vi "FCE_TS_Action_WriteChannelNames.vi"() -> ()   [LabVIEW 2017]
uses:
  FCE_TS_FGlob_V001.llb/FCE_TS_FGlob_TDefEnumcDAQDIItems.ctl
  FCE_TS_FGlob_V001.llb/FCE_TS_FGlob_TDefEnumcDAQDOItems.ctl
  FCE_TS_FGlob_V001.llb/FCE_TS_FGlob_TDefEnumcDAQAIItems.ctl
  FCE_TS_FGlob_V001.llb/FCE_TS_FGlob_TDefEnumcDAQAOItems.ctl
  FCE_TS_FGlob_V001.llb/FCE_TS_FGlob_TDefEnumCANReadItems.ctl
panel:
  in  "Tab Control":enum32{"DI", "DO", "AI", "AO", "CAN"}(tab)
  in  "PCI DI Item":T1
  out "Signal Name":string[](array[string])=["EK_TS", "EZ_Um1", "EZ_Um2", "EZ_Um3", "WZ_TS", "NP", "LP", "HP", "ROP", "CO2P", "WP", "EZ_IW", "ESTB_LB", "ESTB_HB", "ESTB_WB", "ESTB_H1", "WZ_Pu", "KWZ_St", "KL_LAB", "KL_HAB", "KWLo_WB", "KWLu_WB", "WLo_LB", "WLu_LB", "WLo_HB", "WLu_HB", "EZ_TK1-3", "Res_5", "Res_4", "Res_3", "Res_2", "Res_1"]
  out "Signal Name":string[](array[string])
  in  "PCI DO Item":T2
  out "Signal Name":string[](array[string])=["AI0", "AI1", "AI2", "AI3"]
  in  "PCI AI Item":T3=enum."Fp_So_TS"
  out "Signal Name":string[](array[string])=["AO0", "AO1", "AO2", "AO3"]
  in  "PCI AO Item":T4
  out "Signal Name CAN":string[](array[string])=["F_P_H_SI", "F_T_S_0"]
  in  "CAN Read Items":T5
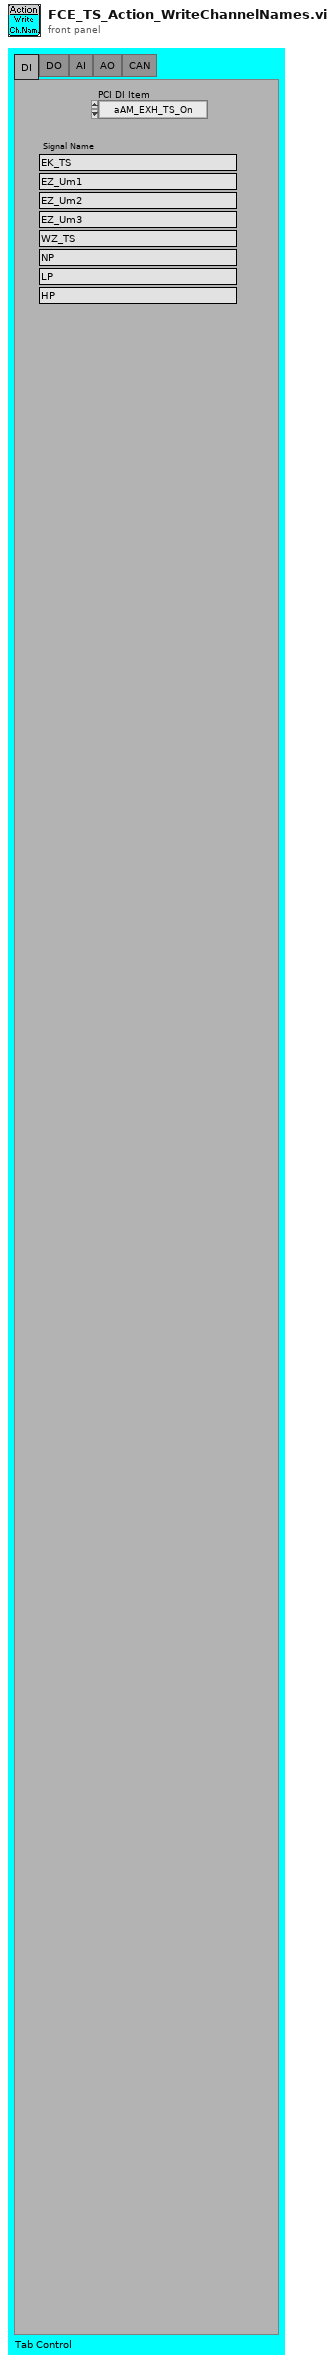
[diagram p1: front panel]
types:
  T1 = typedef "FCE_TS_FGlob_TDefEnumcDAQDIItems.ctl" = enum16{"aAM_EXH_TS_On", "Adp_EXH_TS_Off", "Adp_EXH_TS_On", "HcH_TS_Warn", "HcH_TS_Alarm", "Reserve_DI_2_0_5", "Reserve_DI_2_0_6", "Reserve_DI_2_0_7"}
  T2 = typedef "FCE_TS_FGlob_TDefEnumcDAQDOItems.ctl" = enum16{"aFY_OTV_TS1", "aFY_OTV_TS2", "aFY_EXH_TS", "aEK_SRC_TS", "Reserve_DO_3_0_4", "Reserve_DO_3_0_5", "Reserve_DO_3_0_6", "Reserve_DO_3_0_7"}
  T3 = typedef "FCE_TS_FGlob_TDefEnumcDAQAIItems.ctl" = enum16{"Fp_HPRU_TS1", "Fp_HPRU_TS2", "Fp_So_TS", "AT_EXH_TS", "EU_DCDCi_TS", "EI_DCDC24V_TS", "EI_DIV25A_TS", "EI_DCDC12V_TS", "EI_ETC_TS", "EI_DIV40A_TS", "EI_DCDCi_TS", "EI_DCDCo_TS", "EI_BAT_TS", "EI_LOAD_TS", "Reserve_AI_4_2", "Reserve_AI_4_3", "AT_Si_TS", "AT_So_TS", "CT_Si_TS", "CT_So_TS", "Ck_CP1i_TS", "Cp_CP1i_TS", "Cp_CP1o_TS", "Cp_CP2o_TS"}
  T4 = typedef "FCE_TS_FGlob_TDefEnumcDAQAOItems.ctl" = enum16{"Dummy_AO"}
  T5 = typedef "FCE_TS_FGlob_TDefEnumCANReadItems.ctl" = enum16{"F_P_H_SI_0", "F_T_S_0_0", "F_T_S_opt_0", "F_I_S_0", "F_CH_A_VO_0", "State_F_R_S_In_0", "State_F_SV_H_Si_0", "State_F_SV_H_So_0", "Purge_Time_0", "F_SV_H_SI_0", "F_R_S_0", "F_SV_H_So_0", "F_GP_A1_0", "F_GP_A2_0", "F_U_S_0", "F_RPM_V_0", "State_Set_EA_L0_0", "State_EA_L0_0", "State_EA_L1_0", "F_P_H_SI_1", "F_T_S_0_1", "F_T_S_opt_1", "F_I_S_1", "F_CH_A_VO_1", "State_F_R_S_In_1", "State_F_SV_H_Si_1", "State_F_SV_H_So_1", "Purge_Time_1", "F_SV_H_SI_1", "F_R_S_1", "F_SV_H_So_1", "F_GP_A1_1", "F_GP_A2_1", "F_U_S_1", "F_RPM_V_1", "State_Set_EA_L0_1", "State_EA_L0_1", "State_EA_L1_1", "F_P_H_SI_2", "F_T_S_0_2", "F_T_S_opt_2", "F_I_S_2", "F_CH_A_VO_2", "State_F_R_S_In_2", "State_F_SV_H_Si_2", "State_F_SV_H_So_2", "Purge_Time_2", "F_SV_H_SI_2", "F_R_S_2", "F_SV_H_So_2", "F_GP_A1_2", "F_GP_A2_2", "F_U_S_2", "F_RPM_V_2", "State_Set_EA_L0_2", "State_EA_L0_2", "State_EA_L1_2", "F_P_H_SI_3", "F_T_S_0_3", "F_T_S_opt_3", "F_I_S_3", "F_CH_A_VO_3", "State_F_R_S_In_3", "State_F_SV_H_Si_3", "State_F_SV_H_So_3", "Purge_Time_3", "F_SV_H_SI_3", "F_R_S_3", "F_SV_H_So_3", "F_GP_A1_3", "F_GP_A2_3", "F_U_S_3", "F_RPM_V_3", "State_Set_EA_L0_3", "State_EA_L0_3", "State_EA_L1_3", "F_P_H_SI_4", "F_T_S_0_4", "F_T_S_opt_4", "F_I_S_4", "F_CH_A_VO_4", "State_F_R_S_In_4", "State_F_SV_H_Si_4", "State_F_SV_H_So_4", "Purge_Time_4", "F_SV_H_SI_4", "F_R_S_4", "F_SV_H_So_4", "F_GP_A1_4", "F_GP_A2_4", "F_U_S_4", "F_RPM_V_4", "State_Set_EA_L0_4", "State_EA_L0_4", "State_EA_L1_4", "F_P_H_SI_5", "F_T_S_0_5", "F_T_S_opt_5", "F_I_S_5", "F_CH_A_VO_5", "State_F_R_S_In_5", "State_F_SV_H_Si_5", "State_F_SV_H_So_5", "Purge_Time_5", "F_SV_H_SI_5", "F_R_S_5", "F_SV_H_So_5", "F_GP_A1_5", "F_GP_A2_5", "F_U_S_5", "F_RPM_V_5", "State_Set_EA_L0_5", "State_EA_L0_5", "State_EA_L1_5", "F_P_H_SI_6", "F_T_S_0_6", "F_T_S_opt_6", "F_I_S_6", "F_CH_A_VO_6", "State_F_R_S_In_6", "State_F_SV_H_Si_6", "State_F_SV_H_So_6", "Purge_Time_6", "F_SV_H_SI_6", "F_R_S_6", "F_SV_H_So_6", "F_GP_A1_6", "F_GP_A2_6", "F_U_S_6", "F_RPM_V_6", "State_Set_EA_L0_6", "State_EA_L0_6", "State_EA_L1_6", "C_P_R_CAN_0", "C_U_E_CAN_0", "Initalisierung", "Stand_By", "Rack_Start", "Rack_In_Betrieb", "Rack_Shut_Down", "System_WARN", "System_EPO", "C_SV_H_T", "C_R_L", "C_R_R", "C_I_L_Set", "C_SV_H_R", "C_RPM_V_R", "C_T_A_R", "C_I_L", "C_p_H_Ri", "C_p_H_Ro", "C_p_H_T"}
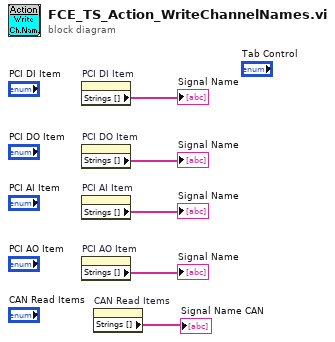
[diagram p0: block diagram]
diagram:
  n1 = property on="PCI DI Item" class="Enum (strikt)"() -> ("Strings []"=→"Signal Name":string[])  [unwired: 2 in, 2 out]
  n2 = property on="PCI DO Item" class="Enum (strikt)"() -> ("Strings []"=→"Signal Name":string[])  [unwired: 2 in, 2 out]
  n3 = property on="PCI AI Item" class="Enum (strikt)"() -> ("Strings []"=→"Signal Name":string[])  [unwired: 2 in, 2 out]
  n4 = property on="PCI AO Item" class="Enum (strikt)"() -> ("Strings []"=→"Signal Name":string[])  [unwired: 2 in, 2 out]
  n5 = property on="CAN Read Items" class="Enum (strikt)"() -> ("Strings []"=→"Signal Name CAN":string[])  [unwired: 2 in, 2 out]
